vi "FindPicturesFolderFromRawData.vi"(11 "RawDataFile":path) -> (0 "SurreyPath?":bool, 1 "RawDataName":string, 2 "PicturesPath":path)   [LabVIEW 2015]
doc: "Finds the location of the Pictures folder for a given RawDataFile"
panel:
  # "Finds the location of the Pictures folder for a given RawDataFile"
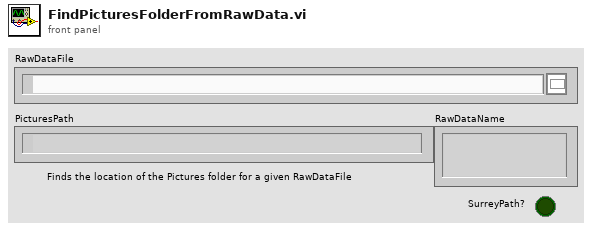
[diagram p1: front panel]
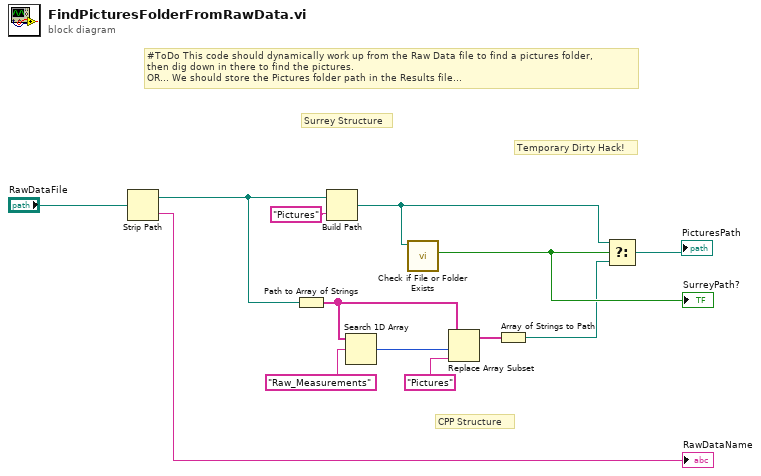
[diagram p0: block diagram]
diagram:
  # "#ToDo This code should dynamically work up from the Raw Data file to find a pictures folder, \nthen dig down in there to find the pictures.\nOR... We should store the Pictures folder path in the Results file..."
  # "Temporary Dirty Hack!"
  # "CPP Structure"
  # "Surrey Structure"
  n1 = Strip Path(path="RawDataFile") -> (stripped path=w5:path, name=→"RawDataName":string)
  n2 = Path to Array of Strings(0:w5) -> (2:w7:string[])  [unwired: 1 out]
  n3 = Build Path(base path=w5, name or relative path="Pictures") -> (appended path=w2:path)
  n4 = Search 1D Array(1D array=w7, element="Raw_Measurements") -> (index of element=w8:i32)  [unwired: 1 in]
  n5 = call <vilib>:"Check if File or Folder Exists.vi"("path"=w2) -> ("file or folder exists?"=w4:bool)  [unwired: 8 in, 2 out]
  "SurreyPath?" <- w4
  n6 = Replace Array Subset(array=w7, new element="Pictures", index=w8) -> (w10:string[])
  n7 = Array of Strings to Path(0:w10) -> (2:w3:path)  [unwired: 1 in]
  n8 = Select(t=w2, s=w4, f=w3) -> (s? t:f=→"PicturesPath":path)
